vi "Sequence Micro.vi"(8 "error in (no error)":errorcluster, 10 "Status":string, 11 "Hardware in":refnum<class "Hardware.lvclass">) -> (0 "error out":errorcluster, 3 "Hardware out":refnum<class "Hardware.lvclass">)   [LabVIEW 2020, in "Hardware.lvlib" / "Hardware.lvclass"]
uses:
  Hardware.lvclass
  C:/Program Files (x86)/National Instruments/LabVIEW 2020/vi.lib/ActorFramework/Actor/Actor.lvclass
  <vilib>/ActorFramework/Actor/Actor.lvclass/Actor.ctl
  <vilib>/ActorFramework/Message Enqueuer/Message Enqueuer.lvclass/Message Enqueuer.ctl
  Hardware Messages/Service Micro Msg/Service Micro Msg.lvclass/Service Micro Msg.ctl
  <vilib>/ActorFramework/Message Enqueuer/Init from Existing Queue.vi
  <vilib>/ActorFramework/Message Enqueuer/Enqueue.vi
  Hardware Messages/Service Micro Msg/Service Micro Msg.lvclass
  C:/Program Files (x86)/National Instruments/LabVIEW 2020/vi.lib/ActorFramework/Message/Message.lvclass
  <vilib>/ActorFramework/Message Priority Queue/Priority Enqueue.vi
  <vilib>/ActorFramework/Message Enqueuer/Message Enqueuer.lvclass
  <vilib>/ActorFramework/Actor/Actor.lvclass
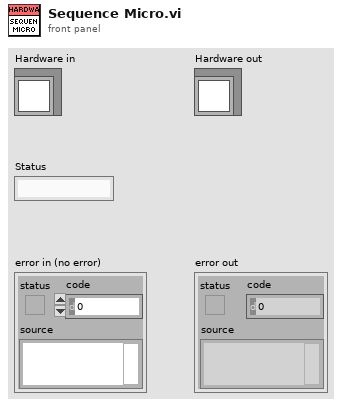
[diagram p1: front panel]
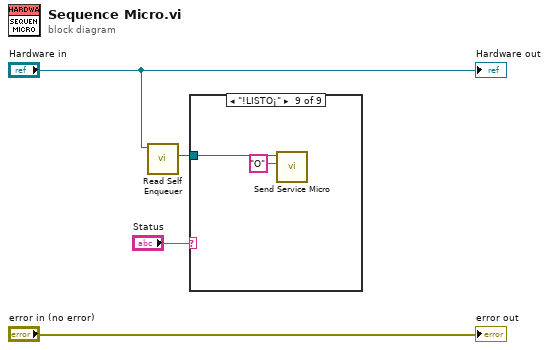
[diagram p0: block diagram]
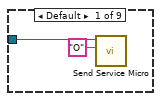
[diagram p2: hidden frame]
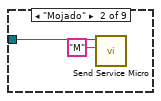
[diagram p3: hidden frame]
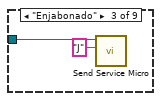
[diagram p4: hidden frame]
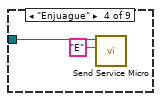
[diagram p5: hidden frame]
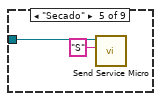
[diagram p6: hidden frame]
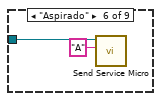
[diagram p7: hidden frame]
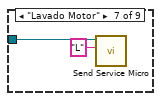
[diagram p8: hidden frame]
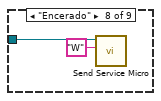
[diagram p9: hidden frame]
diagram:
  n1 = call <vilib>:"Read Self Enqueuer.vi"("Actor"="Hardware in") -> ("Self Enqueuer"=w1:refnum<class "Message Enqueuer.lvclass">)  [unwired: 10 in]
  n2 = case shown="\"!LISTO¡\"" "Status" {
    tunnel: w1 -> [w5 w7 w9 w11 w13 w15 w17 w19 w22]
    frame Default {
      n3 = call "Send Service Micro.vi"("Caracter"="O", "Message Enqueuer"=w5) -> ()  [unwired: 8 in, 2 out]
    }
    frame "Mojado" {
      n4 = call "Send Service Micro.vi"("Caracter"="M", "Message Enqueuer"=w7) -> ()  [unwired: 8 in, 2 out]
    }
    frame "Enjabonado" {
      n5 = call "Send Service Micro.vi"("Caracter"="J", "Message Enqueuer"=w9) -> ()  [unwired: 8 in, 2 out]
    }
    frame "Enjuague" {
      n6 = call "Send Service Micro.vi"("Caracter"="E", "Message Enqueuer"=w11) -> ()  [unwired: 8 in, 2 out]
    }
    frame "Secado" {
      n7 = call "Send Service Micro.vi"("Caracter"="S", "Message Enqueuer"=w13) -> ()  [unwired: 8 in, 2 out]
    }
    frame "Aspirado" {
      n8 = call "Send Service Micro.vi"("Caracter"="A", "Message Enqueuer"=w15) -> ()  [unwired: 8 in, 2 out]
    }
    frame "Lavado Motor" {
      n9 = call "Send Service Micro.vi"("Caracter"="L", "Message Enqueuer"=w17) -> ()  [unwired: 8 in, 2 out]
    }
    frame "Encerado" {
      n10 = call "Send Service Micro.vi"("Caracter"="W", "Message Enqueuer"=w19) -> ()  [unwired: 8 in, 2 out]
    }
    frame "!LISTO¡" {
      n11 = call "Send Service Micro.vi"("Caracter"="O", "Message Enqueuer"=w22) -> ()  [unwired: 8 in, 2 out]
    }
  }
  "error out" <- "error in (no error)"
  "Hardware out" <- "Hardware in"
